vi "Get Doc Object from UID[].vi"(0 "LV MDI":refnum<class "LV MDI.lvclass">, 5 "Doc ÙID[]":string[](array[string]), 11 "error in":errorcluster) -> (4 "LV MDI":refnum<class "LV MDI.lvclass">, 6 "Doc obj[]":refnum<class "Document.lvclass">[](array[class]), 8 "Doc index[]":i32[](array[numeric]), 15 "error Out":errorcluster)   [LabVIEW 2016, in "LV MDI.lvclass"]
uses:
  LV MDI.lvclass
  Document/Document base/Document.lvclass
  LV MDI.lvclass/LV MDI.ctl
  Document/Document base/Document.lvclass/Document.ctl
  Document/Document base/property/Read Doc UID.vi
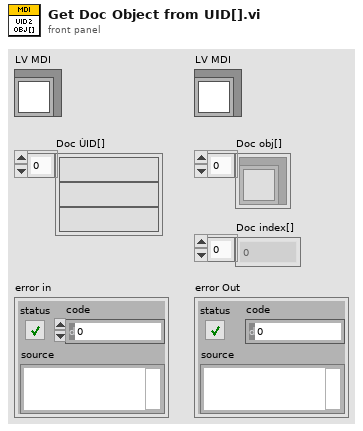
[diagram p1: front panel]
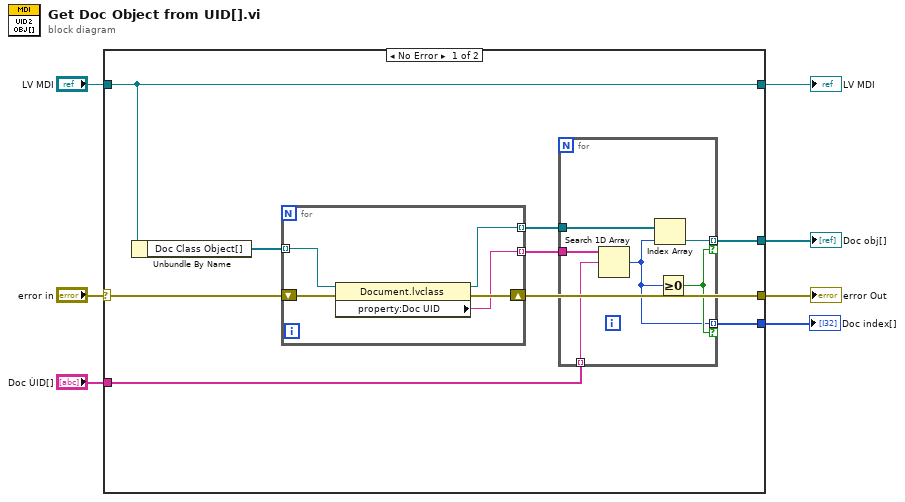
[diagram p0: block diagram]
diagram:
  n1 = case shown="No Error" "error in" {
    selector: "error in" -> [w15 w29]
    tunnel: "Doc ÙID[]" -> [w16 _]
    tunnel: [w14 w29] -> w5
    tunnel: [w13 _] -> w4
    tunnel: "LV MDI" -> [w9 w28]
    tunnel: [w9 w28] -> w2
    tunnel: [w8 _] -> w1
    frame No Error {
      n2 = Unbundle By Name(w9) -> ("Doc Class Object[]"=w12:refnum<class "Document.lvclass">[])
      n3 = for {
        tunnel: w12 -> [w25] mode=indexing
        shift-right: [w26] -> w14
        shift-left: w15 -> [w27]
        tunnel: [w23] -> w10 mode=indexing
        tunnel: [w24] -> w11 mode=indexing
        n4 = property class="Document.lvclass"(reference=w25, error in=w27) -> (reference out=w24:refnum<class "Document.lvclass">, error out=w26:errorcluster, "property:Doc UID"=w23:string)
      }
      n5 = for {
        tunnel: w11 -> [w20]
        tunnel: w10 -> [w22]
        tunnel: w16 -> [w21] mode=indexing
        tunnel: [w19] -> w13 mode=indexing if=w18
        tunnel: [w17] -> w8 mode=indexing if=w18
        n6 = Search 1D Array(1D array=w22, element=w21) -> (index of element=w17:i32)  [unwired: 1 in]
        n7 = Index Array(array=w20, index=w17) -> (element=w19:refnum<class "Document.lvclass">)
        n8 = Greater Or Equal To 0?(x=w17) -> (x >= 0?=w18:bool)
      }
    }
    frame Error {
    }
  }
  "error Out" <- w5
  "Doc obj[]" <- w4
  "LV MDI" <- w2
  "Doc index[]" <- w1
